vi "Hello.vi"(7 "LabVIEW Web Service Request":refnum<class "Web Request.lvclass">) -> ()   [LabVIEW 2014]
uses:
  <vilib>/wsapi/Web Request.lvclass
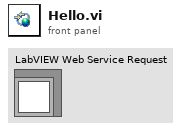
[diagram p1: front panel]
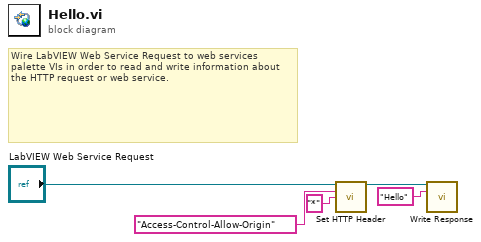
[diagram p0: block diagram]
diagram:
  # "Wire LabVIEW Web Service Request to web services palette VIs in order to read and write information about the HTTP request or web service."
  n1 = call <vilib>:"Set HTTP Header.vi"("LabVIEW Web Service Request"="LabVIEW Web Service Request", "header"="Access-Control-Allow-Origin", "header value"="*") -> ("LabVIEW Web Service Request out"=w1:refnum<class "Web Request.lvclass">)  [unwired: 11 in, 1 out]
  n2 = call <vilib>:"Write Response.vi"("LabVIEW Web Service Request"=w1, "response string"="Hello") -> ()  [unwired: 12 in, 2 out]
